vi "SearchSerialNumber.vi"(8 "error in (no error)":errorcluster caption="错误输入（无错误）", 11 "DataBase in":refnum<class "DataBase.lvclass">) -> (0 "error out":errorcluster caption="错误输出", 3 "DataBase out":refnum<class "DataBase.lvclass">)   [LabVIEW 2019, in "DataBase.lvlib" / "DataBase.lvclass"]
uses:
  DataBase.lvclass
  DataBase.lvclass/DataBase.ctl
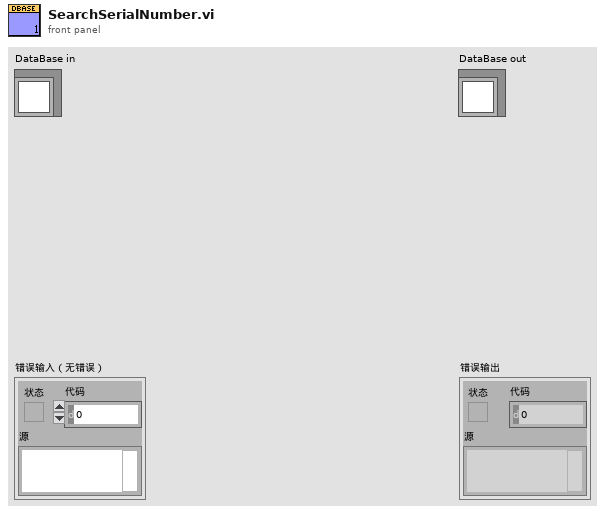
[diagram p1: front panel]
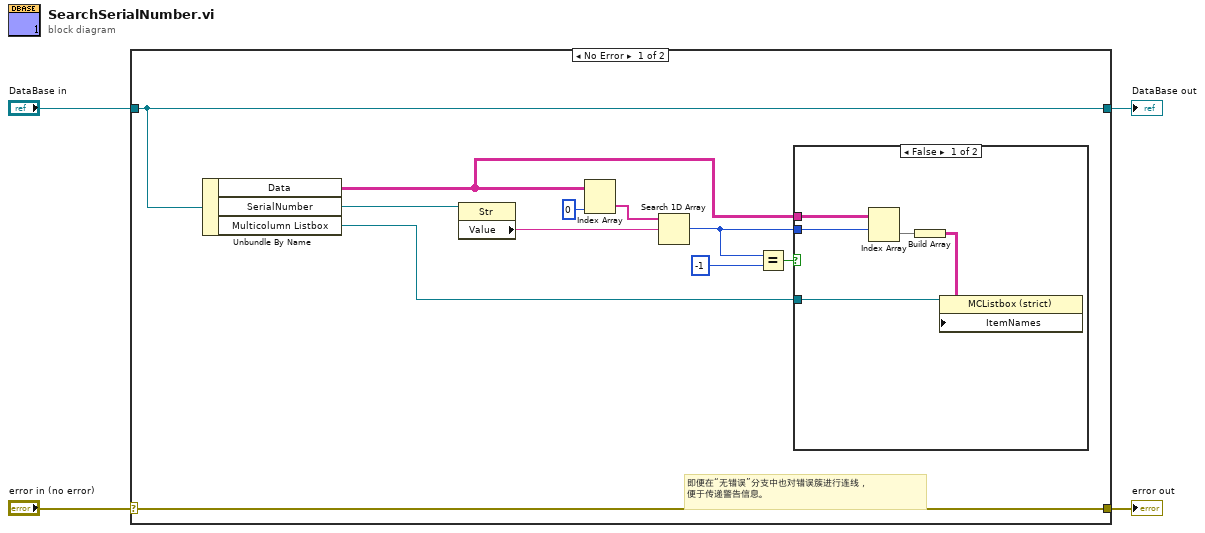
[diagram p0: block diagram]
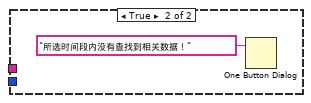
[diagram p2: hidden frame]
diagram:
  n1 = case shown="No Error" "error in (no error)" {
    selector: "error in (no error)" -> [w15 w23]
    tunnel: [w15 w23] -> w3
    tunnel: [w14 w22] -> w1
    tunnel: "DataBase in" -> [w14 w22]
    frame No Error {
      # "即便在“无错误”分支中也对错误簇进行连线，\n便于传递警告信息。"
      n2 = Unbundle By Name(w14) -> ("Data"=w8:string[][], "SerialNumber"=w13:refnum<vi>, "Multicolumn Listbox"=w6:refnum<vi>)
      n3 = property class="Str"(reference=w13) -> ("Value"=w10:string)  [unwired: 1 in, 2 out]
      n4 = Index Array(array=w8, index (col)=0 ("禁用的索引 (列)")) -> (element=w11:string[])  [unwired: 1 in]
      n5 = Search 1D Array(1D array=w11, element=w10) -> (index of element=w7:i32)  [unwired: 1 in]
      n6 = Equal?(x=w7, y=-1) -> (x = y?=w5:bool)
      n7 = case shown="False" w5 {
        tunnel: w8 -> [w20 _]
        tunnel: w7 -> [w19 _]
        tunnel: w6 -> [w18 _]
        frame False {
          n8 = Index Array(array=w20, index (row)=w19) -> (element=w17:string[])  [unwired: 1 in]
          n9 = Build Array(w17) -> (w16:string[][])
          n10 = property class="MCListbox (strict)"(reference=w18, "ItemNames"=w16) -> ()  [unwired: 1 in, 2 out]
        }
        frame True {
          n11 = One Button Dialog(message="所选时间段内没有查找到相关数据！" ("消息")) -> ()  [unwired: 1 in, 1 out]
        }
      }
    }
    frame Error {
    }
  }
  "error out" <- w3
  "DataBase out" <- w1
